vi "RT Host.vi"() -> ()   [LabVIEW 2019]
uses:
  <vilib>/FPGAPlugInAG/cRIO-9039 (Sync)/niLvFpga_Open_cRIO-9039 (Sync).vi
  <vilib>/rvi/interface/common/dynamic/niFpgaDynamicAddResources.vi
  <vilib>/FPGAPlugInAG/Dynamic/niLvFpga_Run_Dynamic.vi
  <vilib>/Utility/error.llb/Error Cluster From Error Code.vi
  <vilib>/RVI Host/nirviSupport.llb/nirviErrorClusterFromErrorCode.vi
  <vilib>/rvi/errors/niLvFpgaAdjustHostInterfaceError.vi
  <userlib>/_OpenG.lib/array/array.llb/Search 1D Array (SGL)__ogtk.vi
  <vilib>/FPGAPlugInAG/Dynamic/niLvFpga_Abort_Dynamic.vi
  <vilib>/FPGAPlugInAG/Dynamic/niLvFpga_Close_Dynamic.vi
  <vilib>/rvi/interface/nirviOpenFPGA/nirviOpenFPGA.xnode
  Bitfiles/cRIO 9039 FPGA Personality.lvbitx
  cRIO FPGA Personality.vi
  <vilib>/rvi/interface/nirviMethod/nirviMethod.xnode
  <vilib>/rvi/interface/nirviCloseFPGA/nirviCloseFPGA.xnode
  <vilib>/measure/NI_MAPro.lvlib
  <vilib>/FPGAPlugInAG/Dynamic/niLvFpga_ReadFifo_Dynamic.vi
  <vilib>/rvi/errors/niLvFpgaMergeErrorWithErrorCode.vi
  <vilib>/measure/matone.llb/Extract Single Tone Information 1 Chan.vi
  <vilib>/rvi/interface/nirviMethod/StockFPGA_InlinedMethodWaitForSingleIRQ.vi
  <vilib>/FPGAPlugInAG/Dynamic/niLvFpga_WaitOnIrq_Dynamic.vi
  <vilib>/FPGAPlugInAG/Dynamic/niLvFpga_AcknowledgeIrq_Dynamic.vi
  <vilib>/FPGAPlugInAG/Dynamic/niLvFpga_WriteFifo_Dynamic.vi
panel:
  out "logical AND":bool
  out "Waveform Graph 2":dbl[](graph)
  out "Waveform Graph 1":dbl[](graph)
  out "error out":errorcluster
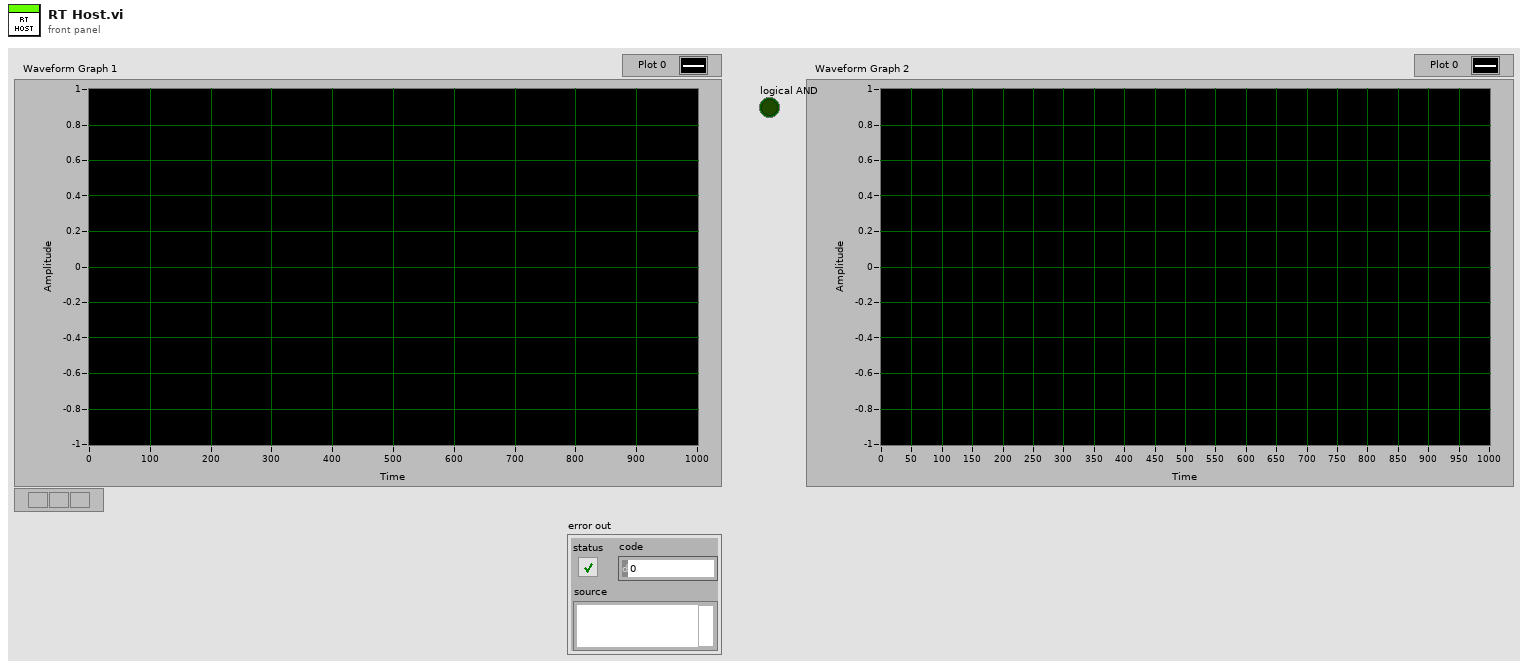
[diagram p1: front panel]
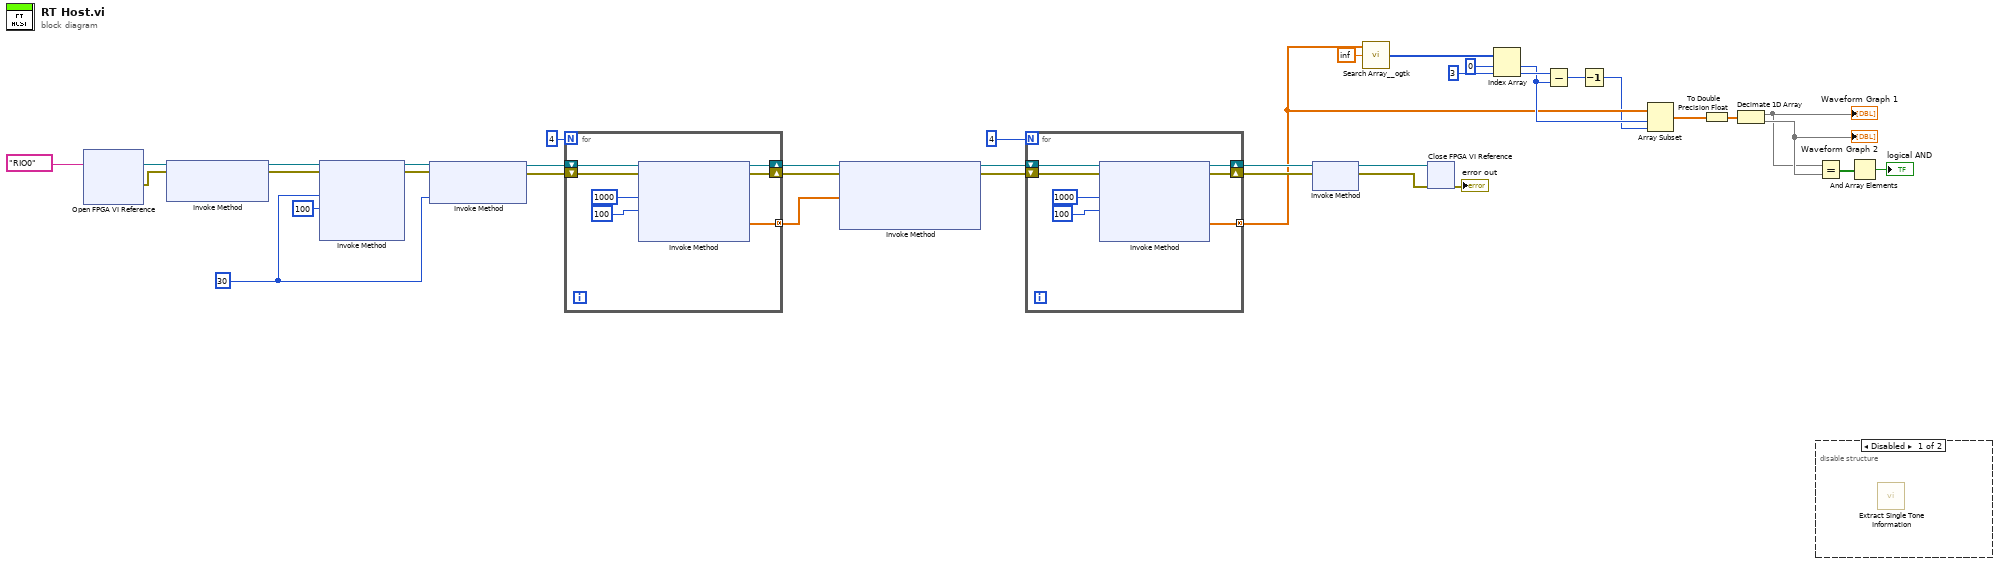
[diagram p0: block diagram]
diagram:
  w36 = 30 ("IRQ Number(s)")
  n1 = xnode "Open FPGA VI Reference"("resource name"=tag "RIO0") -> ("FPGA VI Reference Out"=w27:refnum<k20>, "error out"=w25:errorcluster)  [unwired: 1 in]
  n2 = xnode "Invoke Method"("FPGA VI Reference In"=w27, "error in"=w25) -> ("FPGA VI Reference Out"=w38:refnum<k20>, "error out"=w37:errorcluster)  [unwired: 1 in]
  n3 = xnode "Invoke Method"("FPGA VI Reference In"=w38, "error in"=w37, "IRQ Number(s)"=w36, "Timeout (ms)"=100) -> ("FPGA VI Reference Out"=w35:refnum<k20>, "error out"=w34:errorcluster)  [unwired: 2 out]
  n4 = xnode "Invoke Method"("FPGA VI Reference In"=w35, "error in"=w34, "IRQ Number(s)"=w36) -> ("FPGA VI Reference Out"=w29:refnum<k20>, "error out"=w28:errorcluster)
  n5 = for {
    N: 4 -> [_]
    shift-right: [w41] -> w11
    shift-left: w29 -> [w45]
    shift-right: [w40] -> w7
    shift-left: w28 -> [w44]
    tunnel: [w39] -> w10 mode=concatenating
    n6 = xnode "Invoke Method"("FPGA VI Reference In"=w45, "error in"=w44, "Number of Elements"=u32 1000, "Timeout (ms)"=100) -> ("FPGA VI Reference Out"=w41:refnum<k20>, "error out"=w40:errorcluster, "Data"=w39:sgl[])  [unwired: 1 out]
  }
  n7 = xnode "Invoke Method"("FPGA VI Reference In"=w11, "error in"=w7, "Data"=w10) -> ("FPGA VI Reference Out"=w8:refnum<k20>, "error out"=w6:errorcluster)  [unwired: 1 in, 1 out]
  n8 = for {
    N: 4 -> [_]
    shift-right: [w48] -> w5
    shift-left: w8 -> [w52]
    shift-right: [w47] -> w4
    shift-left: w6 -> [w51]
    tunnel: [w46] -> w3 mode=concatenating
    n9 = xnode "Invoke Method"("FPGA VI Reference In"=w52, "error in"=w51, "Number of Elements"=u32 1000, "Timeout (ms)"=100) -> ("FPGA VI Reference Out"=w48:refnum<k20>, "error out"=w47:errorcluster, "Data"=w46:sgl[])  [unwired: 1 out]
  }
  n10 = xnode "Invoke Method"("FPGA VI Reference In"=w5, "error in"=w4) -> ("FPGA VI Reference Out"=w32:refnum<k20>, "error out"=w31:errorcluster)
  n11 = call-poly <userlib>:"Search Array__ogtk.vi"("Array"=w3, "Element Data"=sgl inf) -> ("Indices of Elements"=w19:i32[])  [unwired: 7 in]
  n12 = xnode "Close FPGA VI Reference"("FPGA VI Reference In"=w32, "error in"=w31) -> ("error out"=→"error out":errorcluster)
  n13 = Index Array(array=w19, index #1=0 ("index"), index #2=3 ("index")) -> (element #1=w15:i32, element #2=w16:i32)
  n14 = Subtract(x=w16, y=w15) -> (x-y=w1:i32)
  n15 = Decrement(x=w1) -> (x-1=w2:i32)
  n16 = Array Subset(array=w3, index=w15, length=w2) -> (w12:sgl[])
  n17 = To Double Precision Float(number=w12) -> (double precision float=w24:dbl[])
  n18 = Decimate 1D Array(w24) -> (w13:dbl[], w14:dbl[])
  "Waveform Graph 1" <- w13
  "Waveform Graph 2" <- w14
  n19 = disable-structure shown="Disabled" {
    frame Disabled {
      n20 = call-poly <vilib>:"Extract Single Tone Information.vi"() -> ()  [unwired: 6 in, 6 out]
    }
    frame Enabled {
    }
  }
  n21 = Equal?(x=w13, y=w14) -> (x = y?=w23:bool[])
  n22 = And Array Elements(Boolean array=w23) -> (logical AND=→"logical AND":bool)
